vi "Create Evaluation String.vi"(8 "error in (no error)":errorcluster, 10 "Evaluation String":string, 11 "Int GT in":refnum<class "Int GT.lvclass">) -> (0 "error out":errorcluster, 3 "Int GT out":refnum<class "Int GT.lvclass">)   [LabVIEW 2018, in "Int GT.lvclass"]
uses:
  Int GT.lvclass
  C:/Users/UKHornP/Documents/Work/Projects/Assert_API/Plugins/Utility/Test Classes/Test.lvclass
  Integer.lvclass
  Test.lvclass
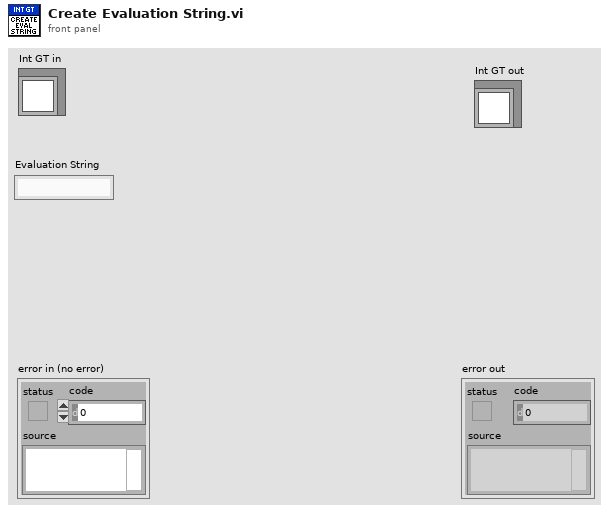
[diagram p1: front panel]
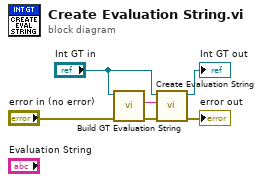
[diagram p0: block diagram]
diagram:
  n1 = call "Build GT Evaluation String.vi"("error in (no error)"="error in (no error)", "Test in"="Int GT in") -> ("error out"=w3:errorcluster, "Equals Evaluation String"=w2:string)  [unwired: 8 in]
  n2 = call-parent "Create Evaluation String.vi"("error in (no error)"=w3, "Evaluation String"=w2, "Integer in"="Int GT in") -> ("error out"=→"error out":errorcluster, "Integer out"=→"Int GT out":refnum<class "Int GT.lvclass">)  [unwired: 7 in]
